vi "subscribe in mapping.vi"(6 "publishing module ID":string, 7 "subscribing module ID":string, 8 "error in":errorcluster, 9 "published element":string, 10 "subscribed element":string, 11 "mappings in":T1) -> (0 "error out":errorcluster, 3 "mappings out":T1)   [LabVIEW 2013, in "engine configuration.lvclass"]
uses:
  engine configuration.lvclass
  simple mapping.ctl
  module channel pairings.ctl
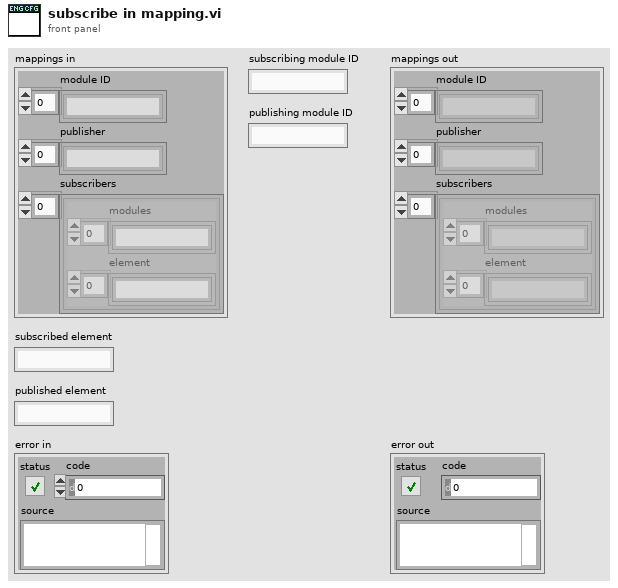
[diagram p1: front panel]
types:
  T1 = typedef "engine configuration.lvclass/simple mapping.ctl" = cluster{"module ID":string[], "publisher":string[], "subscribers":T2[]}
  T2 = typedef "engine configuration.lvclass/module channel pairings.ctl" = cluster{"modules":string[], "element":string[]}
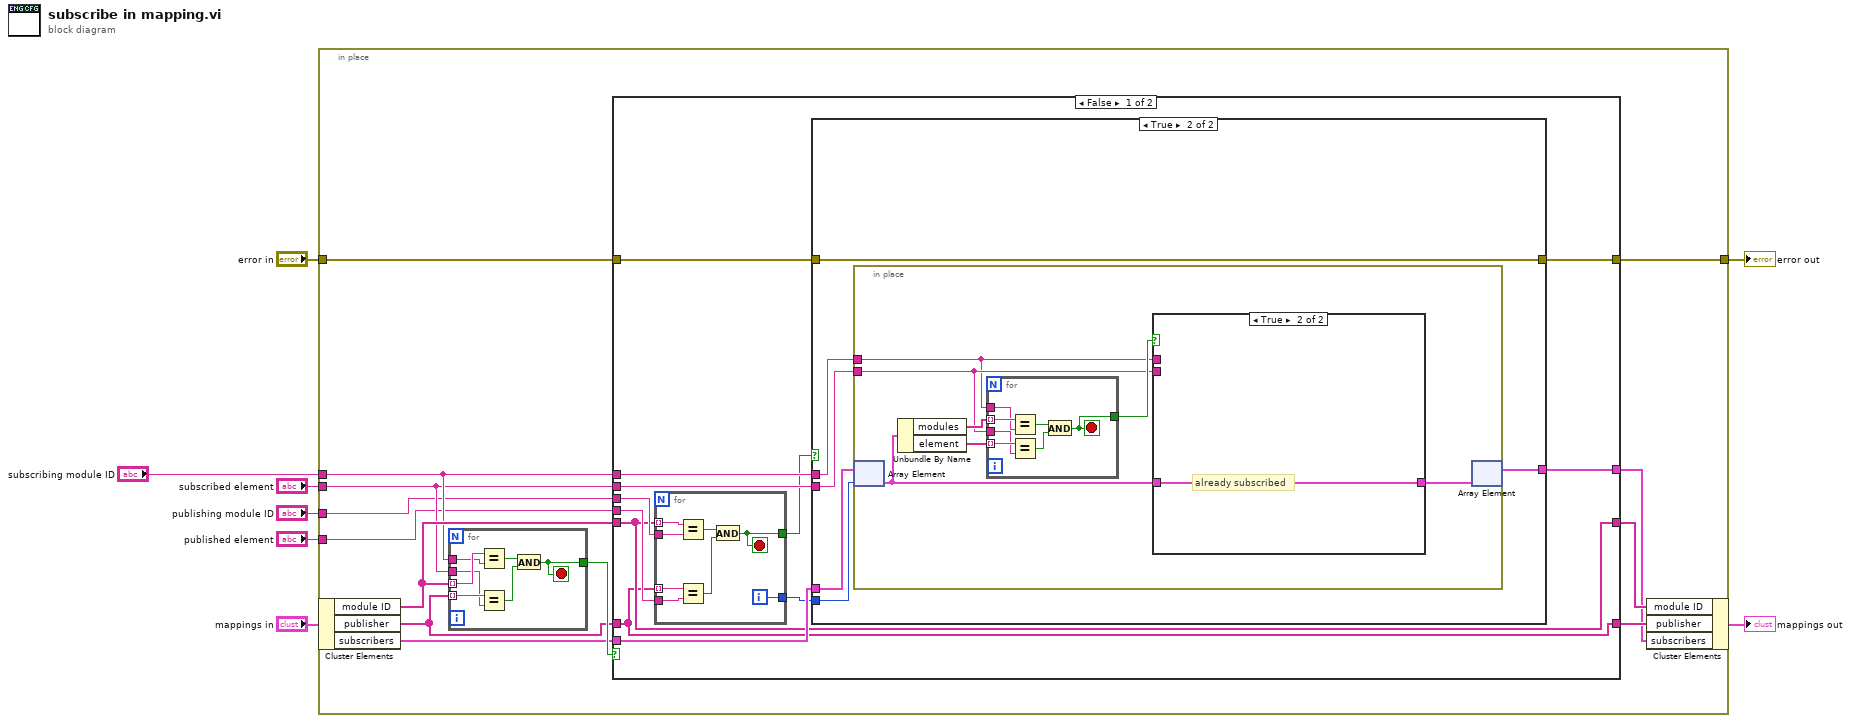
[diagram p0: block diagram]
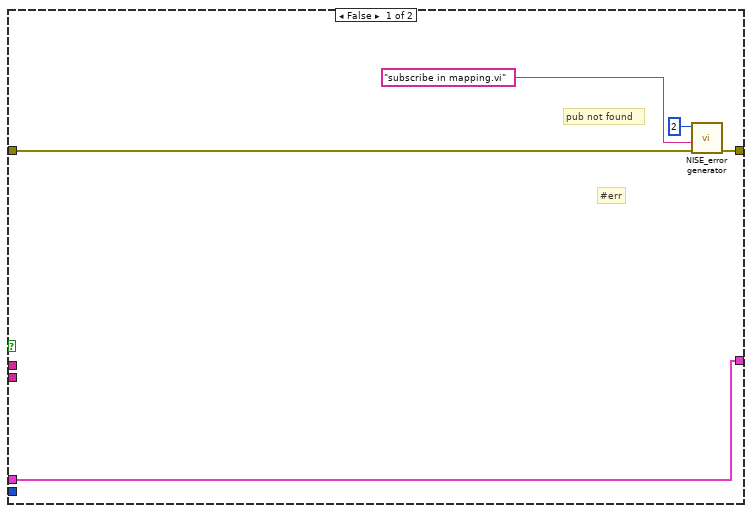
[diagram p2: hidden frame]
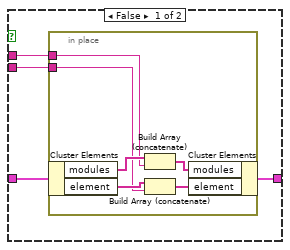
[diagram p3: hidden frame]
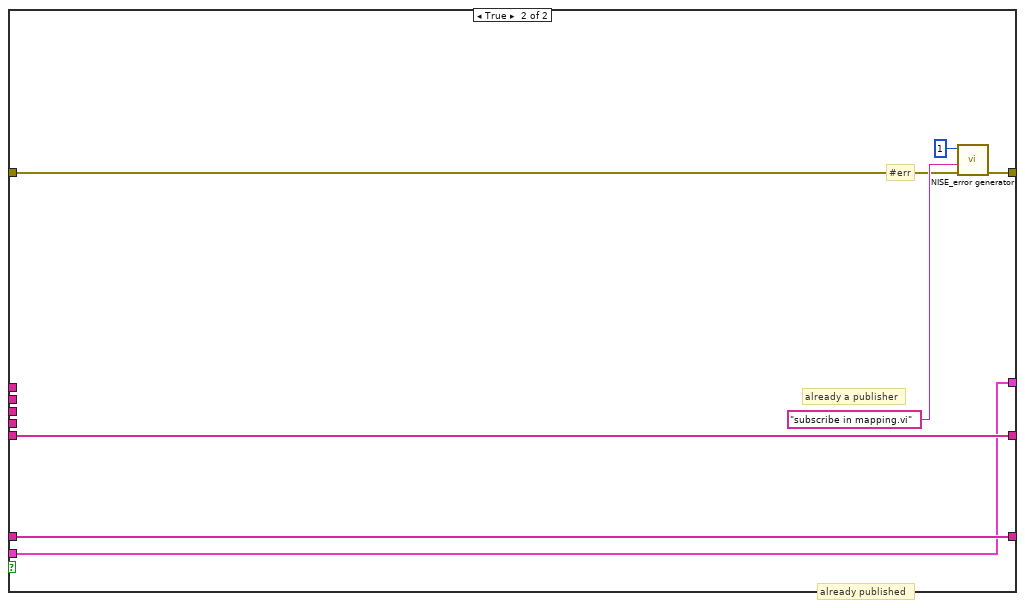
[diagram p4: hidden frame]
diagram:
  n1 = in-place {
    in-place-border: "subscribing module ID" -> [w12]
    in-place-border: "subscribed element" -> [w11]
    in-place-border: [w14] -> w7
    in-place-border: "error in" -> [w13]
    in-place-border: "publishing module ID" -> [w10]
    in-place-border: "published element" -> [w9]
    n2 = in-place-cluster #1("mappings in") -> ("module ID"=w19:string[], "publisher"=w18:string[], "subscribers"=w15:T2[])
    n3 = for {
      tunnel: w19 -> [w91] mode=indexing
      tunnel: w18 -> [w90] mode=indexing
      tunnel: w12 -> [w89]
      tunnel: w11 -> [w88]
      tunnel: [w85] -> w21
      stop <- w85 stop-if-true
      n4 = Equal?(x=w91, y=w89) -> (x = y?=w86:bool)
      n5 = Equal?(x=w90, y=w88) -> (x = y?=w87:bool)
      n6 = And(x=w86, y=w87) -> (x .and. y?=w85:bool)
    }
    n7 = case shown="False" w21 {
      tunnel: [w24 w84] -> w20
      tunnel: w19 -> [w24 w84]
      tunnel: w18 -> [w23 w83]
      tunnel: [w23 w83] -> w17
      tunnel: [w31 w82] -> w16
      tunnel: w15 -> [w30 w82]
      tunnel: [w33 w78] -> w14
      tunnel: w13 -> [w32 w79]
      tunnel: w12 -> [w28 _]
      tunnel: w11 -> [w29 _]
      tunnel: w10 -> [w27 _]
      tunnel: w9 -> [w26 _]
      frame False {
        n8 = for {
          tunnel: [w39] -> w25
          tunnel: w27 -> [w38]
          tunnel: w26 -> [w37]
          tunnel: w24 -> [w36] mode=indexing
          tunnel: w23 -> [w35] mode=indexing
          tunnel: [w34] -> w22
          i -> [w34]
          stop <- w39 stop-if-true
          n9 = Equal?(x=w36, y=w38) -> (x = y?=w40:bool)
          n10 = Equal?(x=w35, y=w37) -> (x = y?=w41:bool)
          n11 = And(x=w40, y=w41) -> (x .and. y?=w39:bool)
        }
        n12 = case shown="True" w25 {
          tunnel: [w45 w52] -> w33
          tunnel: w32 -> [w46 w52]
          tunnel: [w42 w49] -> w31
          tunnel: w30 -> [w42 w50]
          tunnel: w28 -> [_ w47]
          tunnel: w29 -> [_ w48]
          tunnel: w22 -> [_ w51]
          frame False {
            # "pub not found"
            # "#err"
            n13 = call <vilib>:"NISE_error generator.vi"("error in"=w46, "source"="subscribe in mapping.vi", "error code (0)"=2) -> ("error out"=w45:errorcluster)  [unwired: 6 in]
          }
          frame True {
            n14 = in-place {
              in-place-border: w48 -> [w54]
              in-place-border: w47 -> [w53]
              n15 = in-place-array #2(w50, w51) -> (w56:T2)
              n16 = Unbundle By Name(w56) -> ("modules"=w59:string[], "element"=w58:string[])
              n17 = for {
                tunnel: w59 -> [w75] mode=indexing
                tunnel: w58 -> [w74] mode=indexing
                tunnel: w54 -> [w73]
                tunnel: w53 -> [w72]
                tunnel: [w71] -> w57
                stop <- w71 stop-if-true
                n18 = Equal?(x=w75, y=w72) -> (x = y?=w77:bool)
                n19 = Equal?(x=w74, y=w73) -> (x = y?=w76:bool)
                n20 = And(x=w77, y=w76) -> (x .and. y?=w71:bool)
              }
              n21 = case shown="True" w57 {
                tunnel: w56 -> [w63 w70]
                tunnel: [w62 w70] -> w55
                tunnel: w54 -> [w61 _]
                tunnel: w53 -> [w60 _]
                frame False {
                  n22 = in-place {
                    in-place-border: w61 -> [w65]
                    in-place-border: w60 -> [w64]
                    n23 = in-place-cluster #3(w63) -> ("modules"=w69:string[], "element"=w67:string[])
                    n24 = Build Array (concatenate)(w69, w64) -> (w68:string[])
                    n25 = Build Array (concatenate)(w67, w65) -> (w66:string[])
                    n26 = in-place-cluster #3("modules"=w68, "element"=w66) -> (w62:T2)
                  }
                }
                frame True {
                  # "already subscribed"
                }
              }
              n27 = in-place-array #2(w55) -> (w49:T2[])  [unwired: 1 out]
            }
          }
        }
      }
      frame True {
        # "#err"
        # "already a publisher"
        # "already published"
        n28 = call <vilib>:"NISE_error generator.vi"("error in"=w79, "source"="subscribe in mapping.vi", "error code (0)"=1) -> ("error out"=w78:errorcluster)  [unwired: 6 in]
      }
    }
    n29 = in-place-cluster #1("module ID"=w20, "publisher"=w17, "subscribers"=w16) -> (→"mappings out":T1)
  }
  "error out" <- w7
